vi "transferData2UnitFormat.vi"(5 "Data":string[](array[string])) -> (2 "appended array":dbl[][](array[numeric]))   [LabVIEW 2010]
panel:
  out "number":i32[](array[numeric])
  out "测量变量显示":dbl[](array[numeric])
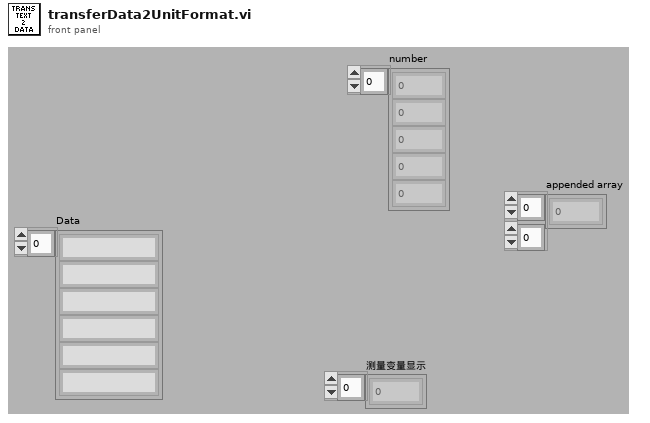
[diagram p1: front panel]
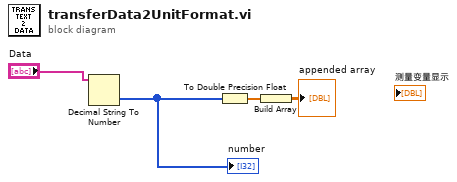
[diagram p0: block diagram]
diagram:
  n1 = Decimal String To Number(string="Data") -> (number=w3:i32[])  [unwired: 2 in, 1 out]
  "number" <- w3
  n2 = To Double Precision Float(number=w3) -> (double precision float=w2:dbl[])
  n3 = Build Array(w2) -> (→"appended array":dbl[][])
